vi "To Test Event.vi"(11 "TestManagerMsg.Assertion in":refnum<class "TestManagerMsg.Assertion.lvclass">) -> (3 "Assert Event Data":T1={"Name"="", "Passed"=FALSE, "Call Chain"=[], "Test Error"={"status"=FALSE, "code"=0, "source"=""}, "Time Stamp"=timestamp(0 s since 1904-01-01), "Unique Assert ID"="", "Test ID"="", "Execution time (s)"=-1.0, "Verbose Explanation"="", "properties"=variant, "measurements"=variant, "limits"=variant})   [LabVIEW 2013, in "Caraya.lvlib" / "TestManagerMsg.Assertion.lvclass"]
uses:
  TestManagerMsg.Assertion.lvclass
  Test Result/Assert Event Data (Extended).ctl
  Test Manager Message/TestManagerMsg.lvclass/TestManagerMsg.ctl
  TestManagerMsg.Assertion.lvclass/TestManagerMsg.Assertion.ctl
  Test Manager Message/TestManagerMsg.lvclass
  Test Result/Test Result.lvclass
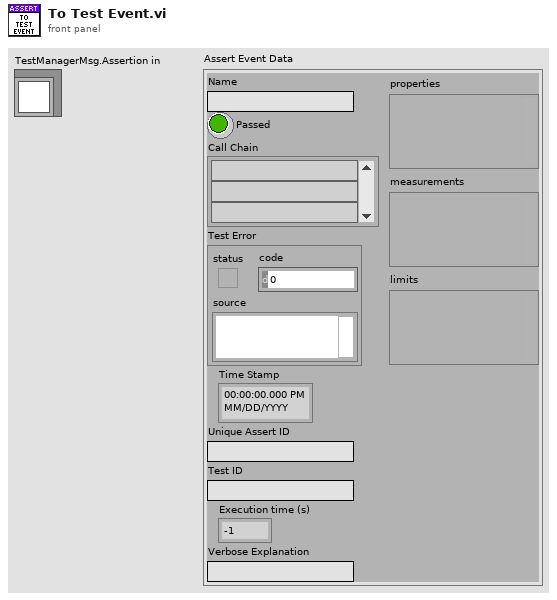
[diagram p1: front panel]
types:
  T1 = typedef "Caraya.lvlib/Test Result.lvclass/Assert Event Data (Extended).ctl" = cluster{"Name":string, "Passed":bool, "Call Chain":string[], "Test Error":errorcluster, "Time Stamp":timestamp, "Unique Assert ID":string, "Test ID":string, "Execution time (s)":dbl, "Verbose Explanation":string, "properties":variant, "measurements":variant, "limits":variant}
  T2 = typedef "Caraya.lvlib/TestManagerMsg.Assertion.lvclass/Assert-Data -- cluster.ctl" = cluster{"Label":string, "Asserted":bool, "call-chain":string[], "upstream-error":errorcluster, "timestamp":timestamp, "Execution time (s)":dbl}
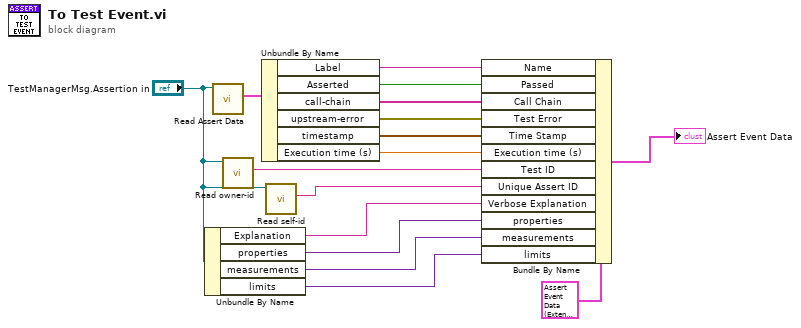
[diagram p0: block diagram]
diagram:
  n1 = Unbundle By Name("TestManagerMsg.Assertion in") -> ("Explanation"=w5:string, "properties"=w4:variant, "measurements"=w3:variant, "limits"=w2:variant)
  n2 = call "Read Assert Data.vi"("Message Assertion"="TestManagerMsg.Assertion in") -> ("Assert Data"=w8:T2)  [unwired: 9 in, 1 out]
  n3 = call "Read owner-id.vi"("TestManagerMsg in"="TestManagerMsg.Assertion in") -> ("owner-id"=w15:string)  [unwired: 9 in, 1 out]
  n4 = Unbundle By Name(w8) -> ("Label"=w9:string, "Asserted"=w13:bool, "call-chain"=w12:string[], "upstream-error"=w11:errorcluster, "timestamp"=w10:timestamp, "Execution time (s)"=w14:dbl)
  n5 = call "Read self-id.vi"("TestManagerMsg in"="TestManagerMsg.Assertion in") -> ("self-id"=w16:string)  [unwired: 9 in, 1 out]
  n6 = Bundle By Name(cluster=T1 {"Name"="", "Passed"=FALSE, "Call Chain"=[], "Test Error"={"status"=FALSE, "code"=0, "source"=""}, "Time Stamp"=timestamp(0 s since 1904-01-01), "Unique Assert ID"="", "Test ID"="", "Execution time (s)"=-1.0, "Verbose Explanation"="", "properties"=variant, "measurements"=variant, "limits"=variant} ("Assert Event Data"), "Name"=w9, "Passed"=w13, "Call Chain"=w12, "Test Error"=w11, "Time Stamp"=w10, "Execution time (s)"=w14, "Test ID"=w15, "Unique Assert ID"=w16, "Verbose Explanation"=w5, "properties"=w4, "measurements"=w3, "limits"=w2) -> (→"Assert Event Data":T1)
